vi "LPos.vi"(0 "reference in":refnum<class "Redis.lvclass">, 1 "Key":string, 5 "Element":string, 7 "Rank(0)":i32, 9 "Count(0)":u32, 11 "Error In":errorcluster, 12 "MaxLength(0)":u32) -> (4 "reference out":refnum<class "Redis.lvclass">, 8 "Positions":u32[](array[numeric]), 15 "Error Out":errorcluster)   [LabVIEW 2020, in "Redis.lvclass"]
doc: "<b>LPOS</b>\n\nThe command returns the index of matching elements inside a Redis list. By default, when no options are given, it will scan the list from head to tail, looking for the first match of \"element\". If the element is found, its index (the zero-based position in the list) is returned. Otherwise, if no match is found, nil is returned.\n\nThe optional arguments and options can modify the command's behavior. The RANK option specifies the \"rank\" of the first element to return, in case there are multiple matches. A rank of 1 means to return the first match, 2 to return the second match, and so forth.\n\nThat is, the second occurrence of \"c\" is at position 6. A negative \"rank\" as the RANK argument tells LPOS to invert the search direction, starting from the tail to the head.\n\nNote that the indexes are still reported in the \"natural\" way, that is, considering the first element starting from the head of the list at index 0, the next element at index 1, and so forth. This basically means that the returned indexes are stable whatever the rank is positive or negative.\n\nWe can combine COUNT and RANK, so that COUNT will try to return up to the specified number of matches, but starting from the Nth match, as specified by the RANK option.\n\nWhen COUNT is used, it is possible to specify 0 as the number of matches, as a way to tell the command we want all the matches found returned as an array of indexes. This is better than giving a very large COUNT option because it is more general.\n\nWhen COUNT is used and no match is found, an empty array is returned. However when COUNT is not used and there are no matches, the command returns nil.\n\nFinally, the MAXLEN option tells the command to compare the provided element only with a given maximum number of list items. So for instance specifying MAXLEN 1000 will make sure that the command performs only 1000 comparisons, effectively running the algorithm on a subset of the list (the first part or the last part depending on the fact we use a positive or negative rank). This is useful to limit the maximum complexity of the command. It is also useful when we expect the match to be found very early, but want to be sure that in case this is not true, the command does not take too much time to run.\n\nWhen MAXLEN is used, it is possible to specify 0 as the maximum number of comparisons, as a way to tell the command we want unlimited comparisons. This is better than giving a very large MAXLEN option because it is more general."
uses:
  Redis.lvclass
  Redis.lvclass/Redis.ctl
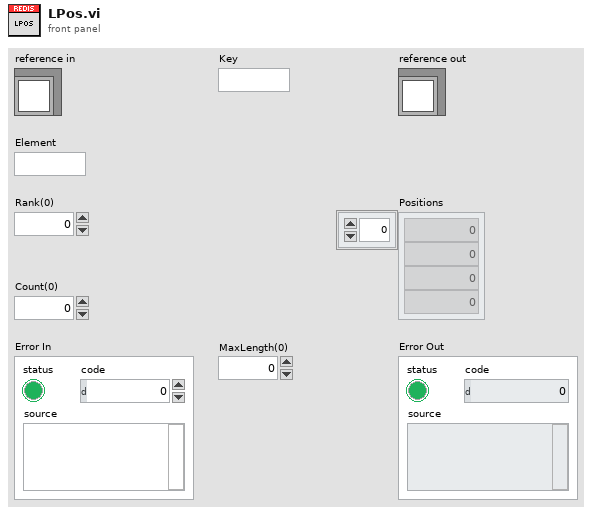
[diagram p1: front panel]
types:
  T1 = typedef "Redis.lvclass/RedisDataType.ctl" = cluster{"Reply Type":T2, "Integer":i64, "String":string, "Multibulk":variant[], "StringData":string[]}
  T2 = typedef "Redis.lvclass/ReplyDataTypeEnum.ctl" = enum16{"None", "Error", "Status", "Nil", "Integer", "String", "Multibulk"}
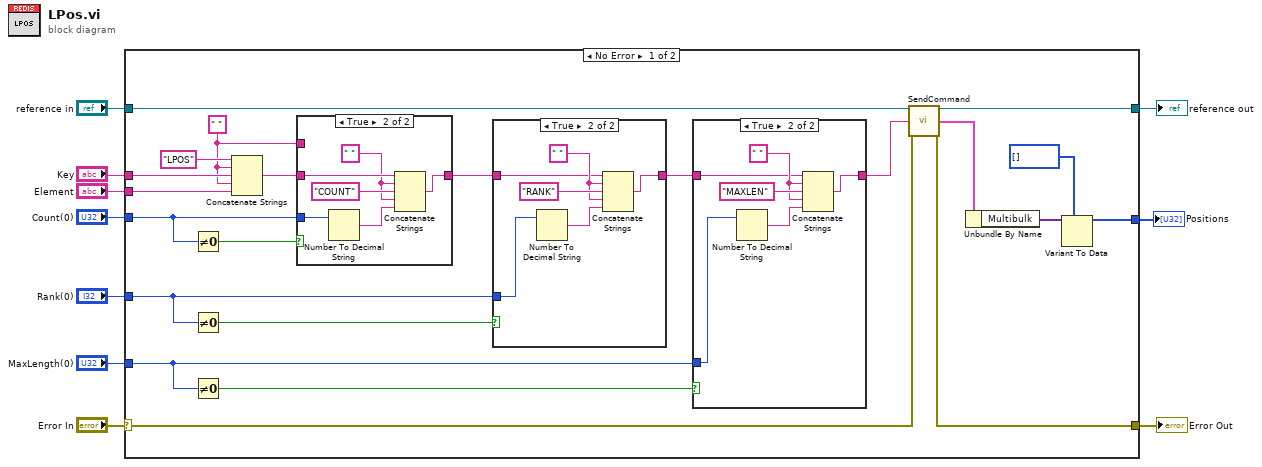
[diagram p0: block diagram]
diagram:
  n1 = case shown="No Error" "Error In" {
    selector: "Error In" -> [w30 w55]
    tunnel: [w29 w55] -> w9
    tunnel: [w32 w54] -> w7
    tunnel: "reference in" -> [w31 w54]
    tunnel: "MaxLength(0)" -> [w16 _]
    tunnel: "Key" -> [w27 _]
    tunnel: "Element" -> [w26 _]
    tunnel: "Count(0)" -> [w22 _]
    tunnel: "Rank(0)" -> [w20 _]
    tunnel: [w11 _] -> w1
    frame No Error {
      w23 = " "
      n2 = Not Equal To 0?(x=w22) -> (x != 0?=w25:bool)
      n3 = Not Equal To 0?(x=w20) -> (x != 0?=w19:bool)
      n4 = Not Equal To 0?(x=w16) -> (x != 0?=w15:bool)
      n5 = Concatenate Strings("LPOS", w23, w27, w23, w26) -> (w24:string)
      n6 = case shown="True" w25 {
        tunnel: w24 -> [w47 w53]
        tunnel: w23 -> [_ _]
        tunnel: w22 -> [_ w51]
        tunnel: [w47 w49] -> w21
        frame False {
        }
        frame True {
          w48 = " "
          n7 = Number To Decimal String(number=w51) -> (decimal integer string=w50:string)  [unwired: 1 in]
          n8 = Concatenate Strings(w53, w48, "COUNT", w48, w50) -> (w49:string)
        }
      }
      n9 = case shown="True" w19 {
        tunnel: w21 -> [w40 w43]
        tunnel: w20 -> [_ w42]
        tunnel: [w40 w41] -> w18
        frame False {
        }
        frame True {
          w44 = " "
          n10 = Number To Decimal String(number=w42) -> (decimal integer string=w45:string)  [unwired: 1 in]
          n11 = Concatenate Strings(w43, w44, "RANK", w44, w45) -> (w41:string)
        }
      }
      n12 = case shown="True" w15 {
        tunnel: w18 -> [w33 w36]
        tunnel: [w33 w35] -> w17
        tunnel: w16 -> [_ w34]
        frame False {
        }
        frame True {
          w37 = " "
          n13 = Number To Decimal String(number=w34) -> (decimal integer string=w38:string)  [unwired: 1 in]
          n14 = Concatenate Strings(w36, w37, "MAXLEN", w37, w38) -> (w35:string)
        }
      }
      n15 = call "SendCommand.vi"("reference in"=w31, "Command"=w17, "Error In"=w30) -> ("reference out"=w32:refnum<class "Redis.lvclass">, "Data"=w14:T1, "Error Out"=w29:errorcluster)  [unwired: 10 in]
      n16 = Unbundle By Name(w14) -> ("Multibulk"=w12:variant[])
      n17 = Variant To Data(type=u32[] [] ("Positions"), Variant=w12) -> (data=w11:u32[])  [unwired: 1 in, 1 out]
    }
    frame Error {
    }
  }
  "Error Out" <- w9
  "reference out" <- w7
  "Positions" <- w1
